vi "Read Totalizer.vi"(7 "Slot Number (1)":u8=1 min=1 max=3 step=1, 8 "error in (no error)":errorcluster, 11 "VISA Resource Name":refnum<visa-resource-name>) -> (0 "error out":errorcluster, 2 "Total":u32, 3 "VISA Resource Name Out":refnum<visa-resource-name>)   [LabVIEW 2012, in "Agilent 34970.lvlib"]
doc: "This VI allows you to read the totalizer on one HP34907 Multifunction module.\n\nThis is an advanced measurment VI. For more information on the different ways to take and configure a measurment, refer to the context help and block diagram of \"HP34970A Advanced Scan Example.vi\"."
uses:
  <instrlib>/Agilent 34970/Agilent 34970.lvlib
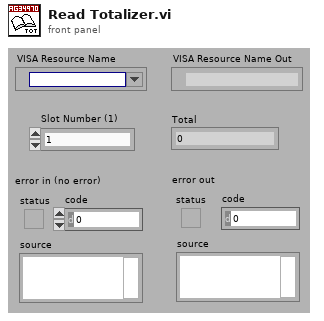
[diagram p1: front panel]
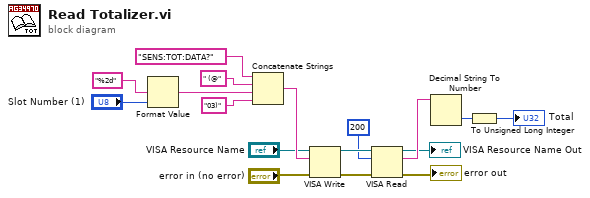
[diagram p0: block diagram]
diagram:
  n1 = Format Value(format string="%2d", value (0)="Slot Number (1)") -> (output string=w5:string)  [unwired: 1 in]
  n2 = Concatenate Strings("SENS:TOT:DATA?", " (@", w5, "03)") -> (w11:string)
  n3 = VISA Write(VISA resource name="VISA Resource Name", write buffer=w11, error in (no error)="error in (no error)") -> (VISA resource name out=w14:refnum<visa-resource-name>, error out=w15:errorcluster)  [unwired: 1 out]
  n4 = VISA Read(VISA resource name=w14, byte count=u32 200 ("byte count (0)"), error in (no error)=w15) -> (VISA resource name out=→"VISA Resource Name Out":refnum<visa-resource-name>, read buffer=w10:string, error out=→"error out":errorcluster)  [unwired: 1 out]
  n5 = Decimal String To Number(string=w10) -> (number=w17:i32)  [unwired: 2 in, 1 out]
  n6 = To Unsigned Long Integer(number=w17) -> (unsigned 32bit integer=→"Total":u32)
